vi "Keithley_data.vi"() -> (0 "String":string)   [LabVIEW 2019]
uses:
  Instrument_Setup.vi
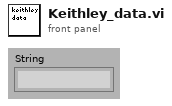
[diagram p1: front panel]
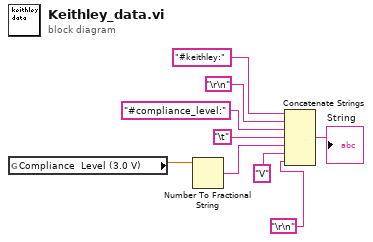
[diagram p0: block diagram]
diagram:
  n1 = global read "Instrument_Setup.vi" "Compliance  Level (3.0 V)"() -> (w4:dbl)
  n2 = Number To Fractional String(number=w4) -> (F-format string=w7:string)  [unwired: 3 in]
  n3 = Concatenate Strings("#keithley:" ("String"), "\r\n", "#compliance_level:" ("String"), "\t", w7, "V" ("String"), "\r\n") -> (→"String":string)
